vi "Read Collection.vi"(8 "error in (no error)":errorcluster, 11 "Test Runner.Collection in":refnum<class "Test Runner.Collection.lvclass">) -> (0 "error out":errorcluster, 2 "Test Runners":refnum<class "Test Runner.lvclass">[](array[class]), 3 "Test Runner.Collection out":refnum<class "Test Runner.Collection.lvclass">)   [LabVIEW 2013, in "Caraya.lvlib" / "Test Runner.Collection.lvclass"]
uses:
  Test Runner.Collection.lvclass
  Test Runner/Test Runner.lvclass
  Test Runner.Collection.lvclass/Test Runner.Collection.ctl
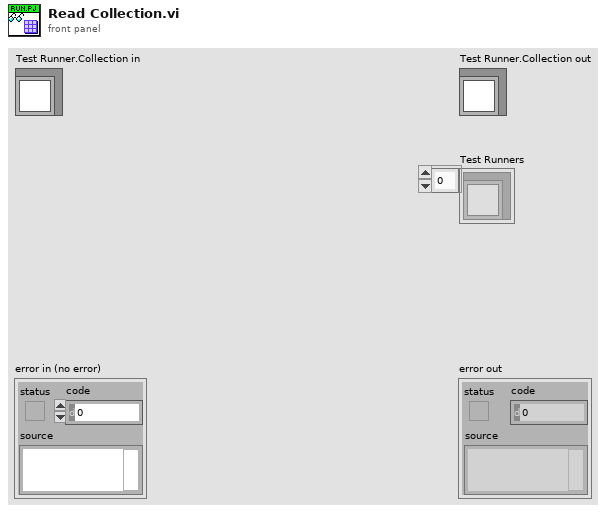
[diagram p1: front panel]
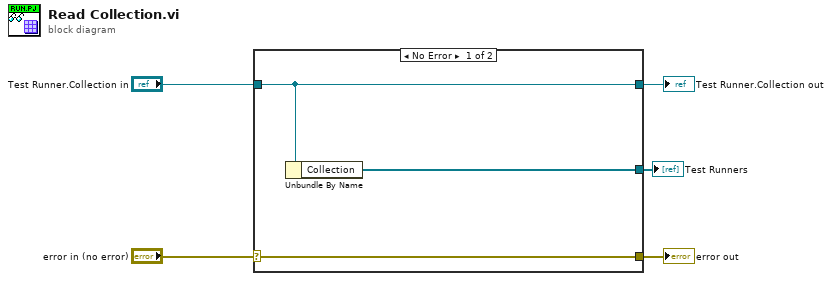
[diagram p0: block diagram]
diagram:
  n1 = case shown="No Error" "error in (no error)" {
    selector: "error in (no error)" -> [w8 w9]
    tunnel: [w8 w9] -> w4
    tunnel: [w7 w10] -> w2
    tunnel: "Test Runner.Collection in" -> [w7 w10]
    tunnel: [w6 _] -> w1
    frame No Error {
      n2 = Unbundle By Name(w7) -> ("Collection"=w6:refnum<class "Test Runner.lvclass">[])
    }
    frame Error {
    }
  }
  "error out" <- w4
  "Test Runner.Collection out" <- w2
  "Test Runners" <- w1
